vi "TestUART.vi"() -> ()   [LabVIEW 2015]
uses:
  <vilib>/rvi/Emulation/niFpgaGetClockAttributes.vi
  <vilib>/rvi/Emulation/niFpgaSctlEmulationGetInTimedLoop.vi
  <vilib>/rvi/Emulation/niFpgaEmulationReportErrorSimple.vi
  <vilib>/rvi/eio/common/nirviEmuTemplateMethod_errors.vi
  <vilib>/rvi/Emulation/niFpgaCriticalErrorInLSC.vi
  <vilib>/eio/EIONode/EIONode.xnode
panel:
  in  "Value":u8
  in  "Baud Rate":u32=80
  out "Real Baud Rate":u32=80
  out "Des BABaus":u32=80
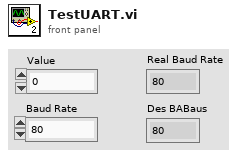
[diagram p1: front panel]
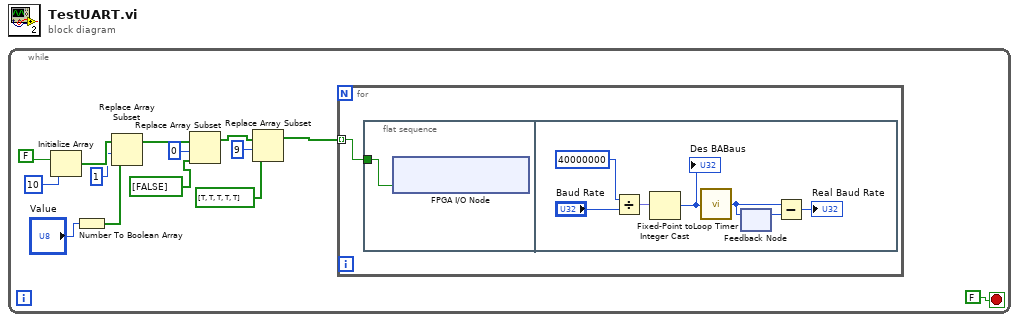
[diagram p0: block diagram]
diagram:
  n1 = while {
    stop <- FALSE stop-if-true
    n2 = Initialize Array(FALSE, i16 10) -> (w11:bool[])
    n3 = Number To Boolean Array(number="Value") -> (Boolean array=w9:bool[])
    n4 = Replace Array Subset(array=w11, new element=w9, index=1) -> (w8:bool[])
    n5 = Replace Array Subset(array=w8, new element=bool[] [FALSE], index=0) -> (w3:bool[])
    n6 = Replace Array Subset(array=w3, new element=bool[] [TRUE, TRUE, TRUE, TRUE, TRUE], index=9) -> (w2:bool[])
    n7 = for {
      tunnel: w2 -> [w15] mode=indexing
      n8 = flat-sequence {
        tunnel: w15 -> [w16]
        frame #0 {
          n9 = xnode "FPGA I/O Node"("Connector1/DIO0"=w16) -> ()  [unwired: 1 in, 1 out]
        }
        frame #1 {
          n10 = Divide(x=40000000, y="Baud Rate") -> (x/y=w18:fxp<+/-,16,16>)
          n11 = Fixed-Point to Integer Cast(1:w18) -> (0:w17:i16)
          "Des BABaus" <- w17
          n12 = call "Loop Timer"("Count(Ticks)"=w17) -> ("Tick Count(Ticks)"=w21:u32)
          n13 = feedback #1() -> (w22:u32)  [unwired: 1 in]
          n14 = feedback-in #1(w21) -> ()
          n15 = Subtract(x=w21, y=w22) -> (x-y=→"Real Baud Rate":u32)
        }
      }
    }
  }
